vi "multicolumn.vi"(0 "LstBox Refnum":refnum<vi>, 1 "Frekanslar":dbl[](array[numeric]), 5 "MCListbox Refnum":refnum<vi>, 7 "Denge Kosulu x2_y2":dbl[][](array[numeric]), 9 "Denge Kosulu x1_x2":dbl[][](array[numeric]), 11 "Denge Kosulu y1_y2":dbl[][](array[numeric]), 12 "frekans index":dbl) -> (4 "Output Denge Kosulu x2_y2":dbl[][](array[numeric]), 6 "Output Denge Kosulu x1_x2":dbl[][](array[numeric]), 8 "Outpu Denge Kosulu y1_y2":dbl[][](array[numeric]))   [LabVIEW 2014]
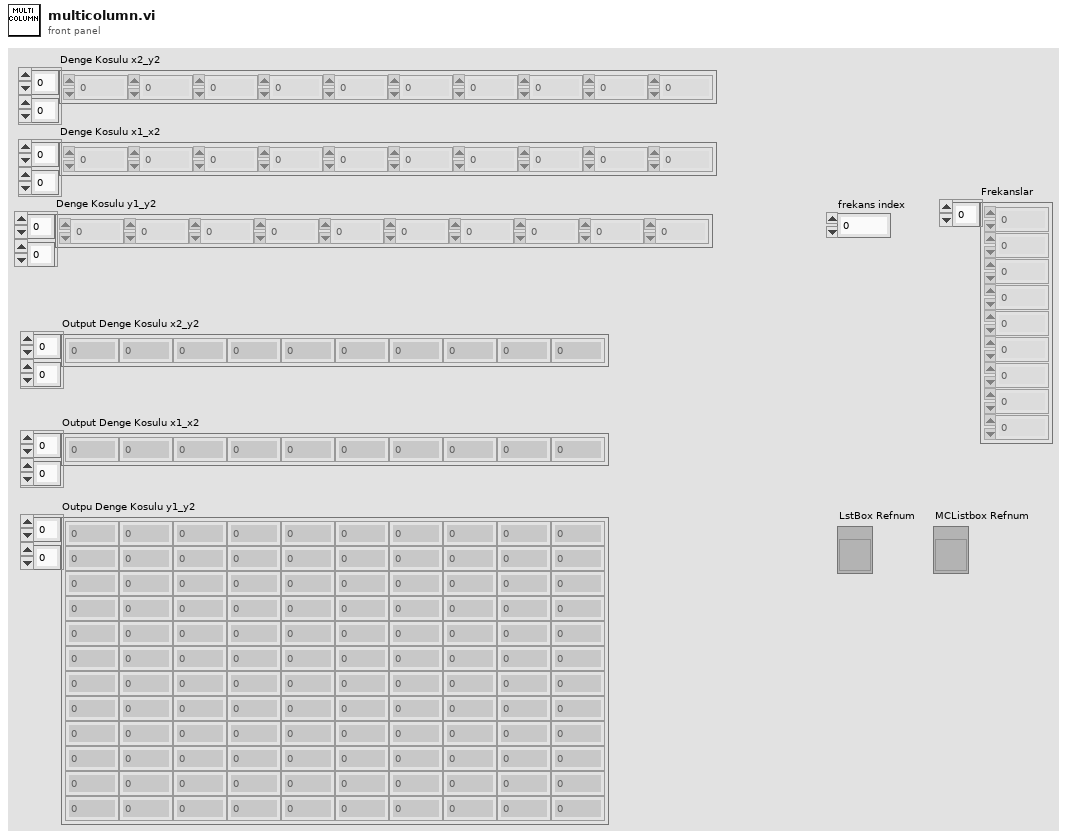
[diagram p1: front panel]
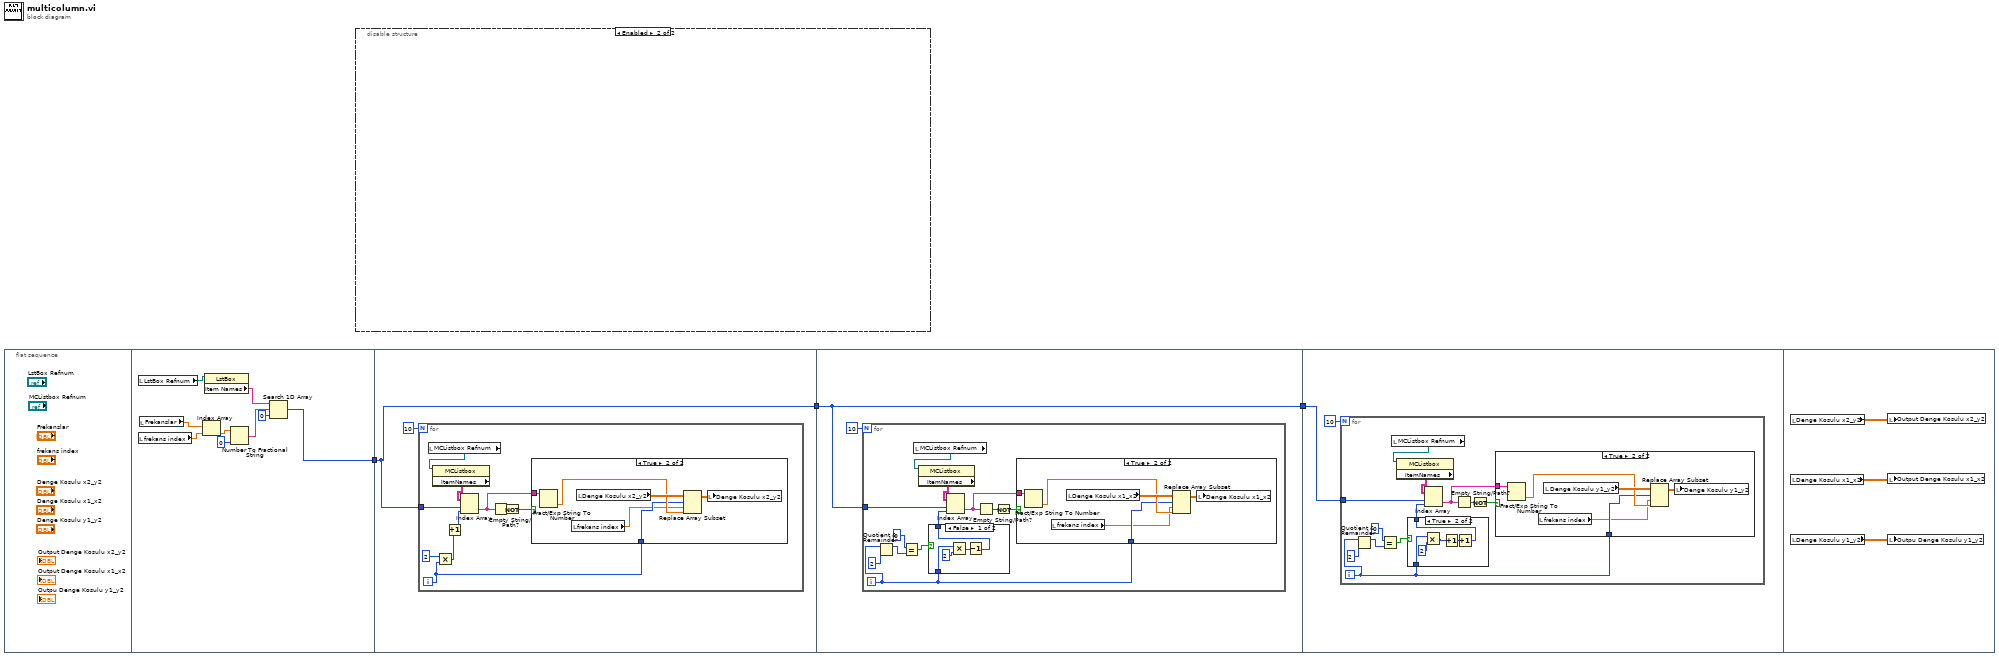
[diagram p0: block diagram]
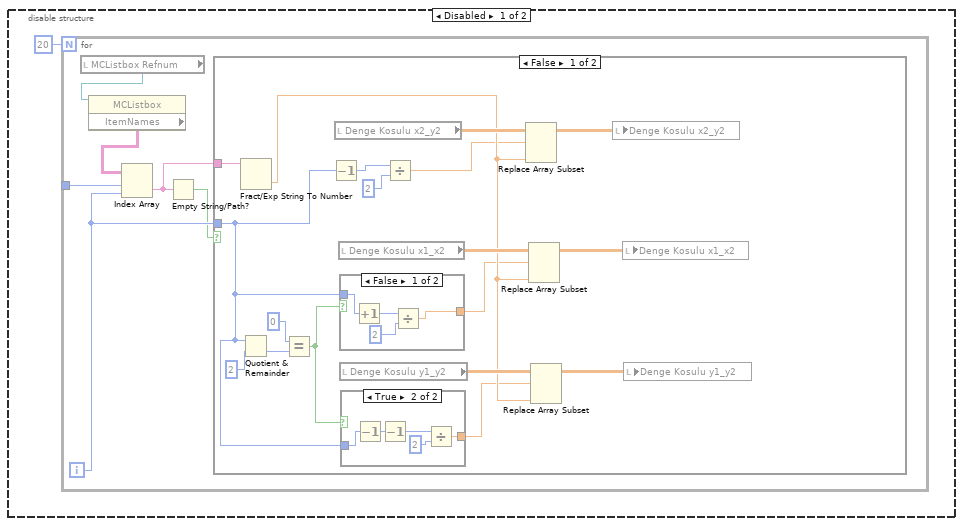
[diagram p2: hidden frame]
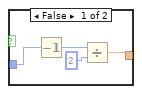
[diagram p3: hidden frame]
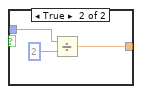
[diagram p4: hidden frame]
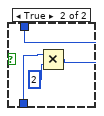
[diagram p7: hidden frame]
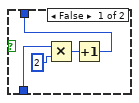
[diagram p9: hidden frame]
diagram:
  n1 = flat-sequence {
    tunnel: [w5] -> w3
    tunnel: w3 -> [w13]
    tunnel: [w13] -> w2
    tunnel: w2 -> [w31]
    tunnel: [w31] -> w1
    tunnel: w1 -> [w58]
    frame #0 {
    }
    frame #1 {
      n2 = local read "LstBox Refnum"() -> (w12:refnum<vi>)
      n3 = local read "frekans index"() -> (w10:dbl)
      n4 = local read "Frekanslar"() -> (w11:dbl[])
      n5 = Index Array(array=w11, index=w10) -> (element=w9:dbl)
      n6 = property class="LstBox"(reference=w12) -> ("Item Names"=w8:string[])  [unwired: 1 in, 2 out]
      n7 = Number To Fractional String(number=w9, precision (6)=i16 0) -> (F-format string=w7:string)  [unwired: 2 in]
      n8 = Search 1D Array(1D array=w8, element=w7, start index (0)=0) -> (index of element=w5:i32)
    }
    frame #2 {
      n9 = for {
        N: 10 -> [_]
        tunnel: w13 -> [w16]
        i -> [w17]
        n10 = local read "MCListbox Refnum"() -> (w24:refnum<vi>)
        n11 = property class="MCListbox"(reference=w24) -> ("ItemNames"=w23:string[][])  [unwired: 1 in, 2 out]
        n12 = Multiply(x=2, y=w17) -> (x*y=w21:i32)
        n13 = Increment(x=w21) -> (x+1=w20:i32)
        n14 = Index Array(array=w23, index (row)=w16, index (col)=w20) -> (element=w18:string)
        n15 = Empty String/Path?(string/path=w18) -> (empty?=w19:bool)
        n16 = Not(x=w19) -> (.not. x?=w15:bool)
        n17 = case shown="True" w15 {
          tunnel: w18 -> [_ w30]
          tunnel: w17 -> [_ w26]
          frame False {
          }
          frame True {
            n18 = Fract/Exp String To Number(string=w30) -> (number=w27:dbl)  [unwired: 3 in, 1 out]
            n19 = local read "frekans index"() -> (w25:dbl)
            n20 = local read "Denge Kosulu x2_y2"() -> (w28:dbl[][])
            n21 = Replace Array Subset(array=w28, new element=w27, index (row)=w26, index (col)=w25) -> (w29:dbl[][])
            n22 = local write "Denge Kosulu x2_y2"(w29) -> ()
          }
        }
      }
    }
    frame #3 {
      n23 = for {
        N: 10 -> [_]
        tunnel: w31 -> [w35]
        i -> [w37]
        n24 = Quotient & Remainder(x=w37, y=2) -> (x-y*floor(x/y)=w33:i32)  [unwired: 1 out]
        n25 = Equal?(x=0, y=w33) -> (x = y?=w38:bool)
        n26 = local read "MCListbox Refnum"() -> (w44:refnum<vi>)
        n27 = property class="MCListbox"(reference=w44) -> ("ItemNames"=w43:string[][])  [unwired: 1 in, 2 out]
        n28 = case shown="False" w38 {
          tunnel: w37 -> [w48 w51]
          tunnel: [w45 w49] -> w36
          frame False {
            n29 = Multiply(x=w48, y=2) -> (x*y=w46:i32)
            n30 = Decrement(x=w46) -> (x-1=w45:i32)
          }
          frame True {
            n31 = Multiply(x=w51, y=2) -> (x*y=w49:i32)
          }
        }
        n32 = Index Array(array=w43, index (row)=w35, index (col)=w36) -> (element=w41:string)
        n33 = Empty String/Path?(string/path=w41) -> (empty?=w42:bool)
        n34 = Not(x=w42) -> (.not. x?=w34:bool)
        n35 = case shown="True" w34 {
          tunnel: w41 -> [_ w57]
          tunnel: w37 -> [_ w53]
          frame False {
          }
          frame True {
            n36 = Fract/Exp String To Number(string=w57) -> (number=w54:dbl)  [unwired: 3 in, 1 out]
            n37 = local read "frekans index"() -> (w52:dbl)
            n38 = local read "Denge Kosulu x1_x2"() -> (w55:dbl[][])
            n39 = Replace Array Subset(array=w55, new element=w54, index (row)=w53, index (col)=w52) -> (w56:dbl[][])
            n40 = local write "Denge Kosulu x1_x2"(w56) -> ()
          }
        }
      }
    }
    frame #4 {
      n41 = for {
        N: 10 -> [_]
        tunnel: w58 -> [w62]
        i -> [w64]
        n42 = Quotient & Remainder(x=w64, y=2) -> (x-y*floor(x/y)=w60:i32)  [unwired: 1 out]
        n43 = Equal?(x=0, y=w60) -> (x = y?=w65:bool)
        n44 = local read "MCListbox Refnum"() -> (w71:refnum<vi>)
        n45 = property class="MCListbox"(reference=w71) -> ("ItemNames"=w70:string[][])  [unwired: 1 in, 2 out]
        n46 = case shown="True" w65 {
          tunnel: w64 -> [w75 w80]
          tunnel: [w72 w76] -> w63
          frame False {
            n47 = Multiply(x=w75, y=2) -> (x*y=w73:i32)
            n48 = Increment(x=w73) -> (x+1=w72:i32)
          }
          frame True {
            n49 = Multiply(x=w80, y=2) -> (x*y=w78:i32)
            n50 = Increment(x=w78) -> (x+1=w77:i32)
            n51 = Increment(x=w77) -> (x+1=w76:i32)
          }
        }
        n52 = Index Array(array=w70, index (row)=w62, index (col)=w63) -> (element=w68:string)
        n53 = Empty String/Path?(string/path=w68) -> (empty?=w69:bool)
        n54 = Not(x=w69) -> (.not. x?=w61:bool)
        n55 = case shown="True" w61 {
          tunnel: w68 -> [_ w86]
          tunnel: w64 -> [_ w82]
          frame False {
          }
          frame True {
            n56 = Fract/Exp String To Number(string=w86) -> (number=w83:dbl)  [unwired: 3 in, 1 out]
            n57 = local read "frekans index"() -> (w81:dbl)
            n58 = local read "Denge Kosulu y1_y2"() -> (w84:dbl[][])
            n59 = Replace Array Subset(array=w84, new element=w83, index (row)=w82, index (col)=w81) -> (w85:dbl[][])
            n60 = local write "Denge Kosulu y1_y2"(w85) -> ()
          }
        }
      }
    }
    frame #5 {
      n61 = local read "Denge Kosulu x2_y2"() -> (w89:dbl[][])
      n62 = local read "Denge Kosulu x1_x2"() -> (w88:dbl[][])
      n63 = local read "Denge Kosulu y1_y2"() -> (w87:dbl[][])
      n64 = local write "Output Denge Kosulu x2_y2"(w89) -> ()
      n65 = local write "Output Denge Kosulu x1_x2"(w88) -> ()
      n66 = local write "Outpu Denge Kosulu y1_y2"(w87) -> ()
    }
  }
  n67 = disable-structure shown="Enabled" {
    frame Disabled {
      n68 = for {
        N: 20 -> [_]
        tunnel: [w95] -> w91
        i -> [w93]
        n69 = local read "MCListbox Refnum"() -> (w97:refnum<vi>)
        n70 = property class="MCListbox"(reference=w97) -> ("ItemNames"=w96:string[][])  [unwired: 1 in, 2 out]
        n71 = Index Array(array=w96, index (row)=w95, index (col)=w93) -> (element=w94:string)
        n72 = Empty String/Path?(string/path=w94) -> (empty?=w92:bool)
        n73 = case shown="False" w92 {
          tunnel: w94 -> [w115 _]
          tunnel: w93 -> [w99 _]
          frame False {
            n74 = Fract/Exp String To Number(string=w115) -> (number=w108:dbl)  [unwired: 3 in, 1 out]
            n75 = Quotient & Remainder(x=w99, y=2) -> (floor(x/y)=w103:i32)  [unwired: 1 out]
            n76 = Equal?(x=0, y=w103) -> (x = y?=w101:bool)
            n77 = Decrement(x=w99) -> (x-1=w107:i32)
            n78 = local read "Denge Kosulu x2_y2"() -> (w114:dbl[][])
            n79 = local read "Denge Kosulu x1_x2"() -> (w113:dbl[][])
            n80 = case shown="False" w101 {
              tunnel: w99 -> [w128 w131]
              tunnel: [w125 w129] -> w100
              frame False {
                n81 = Increment(x=w128) -> (x+1=w127:i32)
                n82 = Divide(x=w127, y=2) -> (x/y=w125:dbl)
              }
              frame True {
                n83 = Divide(x=w131, y=2) -> (x/y=w129:dbl)
              }
            }
            n84 = local read "Denge Kosulu y1_y2"() -> (w112:dbl[][])
            n85 = case shown="True" w101 {
              tunnel: w99 -> [w117 w124]
              tunnel: [w116 w120] -> w98
              frame False {
                n86 = Decrement(x=w117) -> (x-1=w119:i32)
                n87 = Divide(x=w119, y=2) -> (x/y=w116:dbl)
              }
              frame True {
                n88 = Decrement(x=w124) -> (x-1=w123:i32)
                n89 = Decrement(x=w123) -> (x-1=w122:i32)
                n90 = Divide(x=w122, y=2) -> (x/y=w120:dbl)
              }
            }
            n91 = Divide(x=w107, y=2) -> (x/y=w105:dbl)
            n92 = Replace Array Subset(array=w114, new element=w108, index (row)=w105) -> (w111:dbl[][])  [unwired: 1 in]
            n93 = Replace Array Subset(array=w113, new element=w108, index (row)=w100) -> (w110:dbl[][])  [unwired: 1 in]
            n94 = Replace Array Subset(array=w112, new element=w108, index (row)=w98) -> (w109:dbl[][])  [unwired: 1 in]
            n95 = local write "Denge Kosulu x2_y2"(w111) -> ()
            n96 = local write "Denge Kosulu x1_x2"(w110) -> ()
            n97 = local write "Denge Kosulu y1_y2"(w109) -> ()
          }
          frame True {
          }
        }
      }
    }
    frame Enabled {
    }
  }
